vi "Get Current Parameter Value - I32.vi"(7 "Default value":i32, 8 "error in (no error)":errorcluster, 10 "Parameter name":string, 11 "Config in":refnum<class "Config.lvclass">) -> (0 "error out":errorcluster, 2 "Value":i32, 3 "Config out":refnum<class "Config.lvclass">)   [LabVIEW 2026, in "TALOS.lvlib" / "Classes.lvlib" / "Config.lvclass"]
doc: "Get the parameter's value (int) from the currently used configuration. Use the data type terminal to specify the output type."
uses:
  Config.lvclass
  Config.lvclass/Config.ctl
  Get Parameter Value - I32.vi
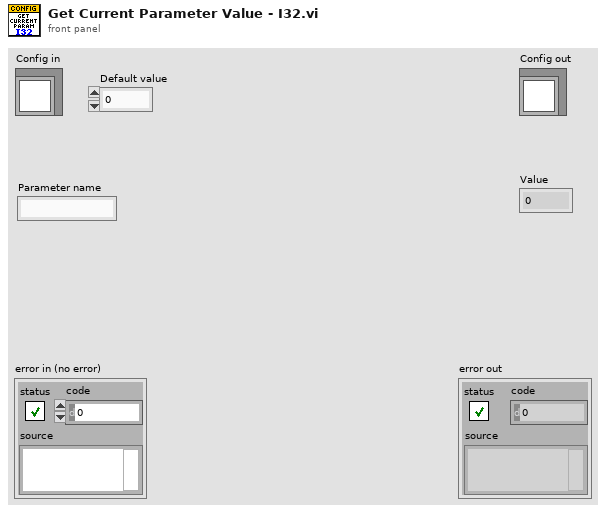
[diagram p1: front panel]
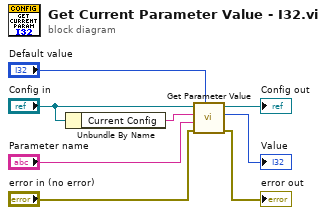
[diagram p0: block diagram]
diagram:
  n1 = Unbundle By Name("Config in") -> ("Current Config"=w6:string)
  n2 = call-poly "Get Parameter Value.vi"("Default value"="Default value", "error in (no error)"="error in (no error)", "Parameter name"="Parameter name", "Config name"=w6, "Config in"="Config in") -> ("error out"=→"error out":errorcluster, "Value"=→"Value":i32, "Config out"=→"Config out":refnum<class "Config.lvclass">)  [unwired: 4 in]
